vi "mecanum encoder read.vi"() -> ()   [LabVIEW 2014]
uses:
  global variables/devrefs.vi
panel:
  out "X Rate":dbl
  out "Y Rate":dbl
  in  "Reset Encoders":bool
  out "Y Distance":dbl
  out "X Distance":dbl
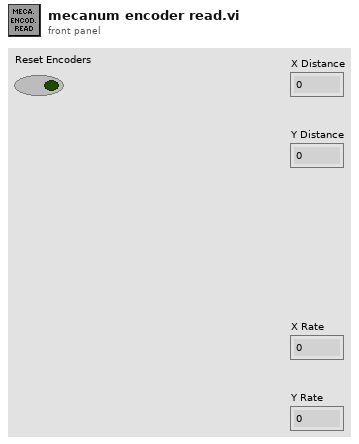
[diagram p1: front panel]
types:
  T1 = typedef "WPI_EncoderDevRef.ctl" = cluster{"DevStatus":errorcluster, "EncoderIndex":T2, "CounterIndex":T3, "DistancePerCount":dbl, "Decoding Type":T4}
  T2 = typedef "FPGA_EncoderIdx.ctl" = enum8{"Enc 0", "Enc 1", "Enc 2", "Enc 3", "Enc 4", "Enc 5", "Enc 6", "Enc 7", "Invalid"}
  T3 = typedef "FPGA_CounterCtrSystemIndex.ctl" = enum8{"Ctr 0", "Ctr 1", "Ctr 2", "Ctr 3", "Ctr 4", "Ctr 5", "Ctr 6", "Ctr 7", "Invalid"}
  T4 = typedef "WPI_EncoderType.ctl" = enum16{"1x", "2x", "4x"}
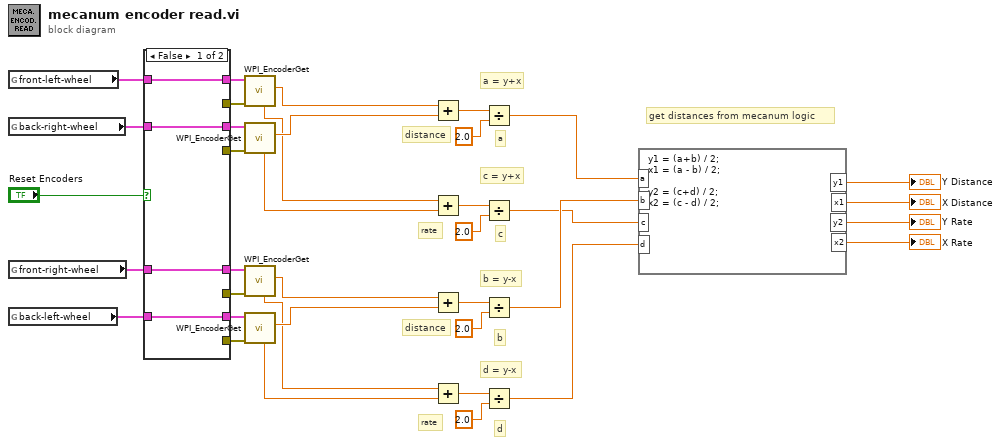
[diagram p0: block diagram]
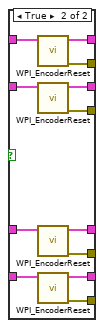
[diagram p2: hidden frame]
diagram:
  # "get distances from mecanum logic"
  # "distance"
  # "distance"
  # "rate"
  # "rate"
  # "c"
  # "c = y+x"
  # "d"
  # "d = y-x"
  # "b"
  # "a"
  # "b = y-x"
  # "a = y+x"
  n1 = global read "devrefs.vi" "front-left-wheel"() -> (w24:T1)
  n2 = global read "devrefs.vi" "back-right-wheel"() -> (w25:T1)
  n3 = global read "devrefs.vi" "front-right-wheel"() -> (w23:T1)
  n4 = global read "devrefs.vi" "back-left-wheel"() -> (w22:T1)
  n5 = case shown="False" "Reset Encoders" {
    tunnel: w25 -> [w40 w49]
    tunnel: w24 -> [w41 w52]
    tunnel: w23 -> [w39 w46]
    tunnel: w22 -> [w38 w43]
    tunnel: [w41 w53] -> w20
    tunnel: [w40 w50] -> w19
    tunnel: [w39 w47] -> w18
    tunnel: [w38 w44] -> w17
    tunnel: [_ w51] -> w16
    tunnel: [_ w48] -> w15
    tunnel: [_ w45] -> w14
    tunnel: [_ w42] -> w13
    frame False {
    }
    frame True {
      n6 = call <vilib>:"WPI_EncoderReset.vi"("EncoderDevRef"=w52) -> ("error out"=w51:errorcluster, "EncoderDevRef"=w53:T1)  [unwired: 9 in]
      n7 = call <vilib>:"WPI_EncoderReset.vi"("EncoderDevRef"=w49) -> ("error out"=w48:errorcluster, "EncoderDevRef"=w50:T1)  [unwired: 9 in]
      n8 = call <vilib>:"WPI_EncoderReset.vi"("EncoderDevRef"=w46) -> ("error out"=w45:errorcluster, "EncoderDevRef"=w47:T1)  [unwired: 9 in]
      n9 = call <vilib>:"WPI_EncoderReset.vi"("EncoderDevRef"=w43) -> ("error out"=w42:errorcluster, "EncoderDevRef"=w44:T1)  [unwired: 9 in]
    }
  }
  n10 = call <vilib>:"WPI_EncoderGet.vi"("error in (no error)"=w16, "EncoderDevRef"=w20) -> ("Distance"=w29:dbl, "Rate"=w6:dbl)  [unwired: 4 in, 4 out]
  n11 = call <vilib>:"WPI_EncoderGet.vi"("error in (no error)"=w15, "EncoderDevRef"=w19) -> ("Distance"=w28:dbl, "Rate"=w5:dbl)  [unwired: 4 in, 4 out]
  n12 = call <vilib>:"WPI_EncoderGet.vi"("error in (no error)"=w14, "EncoderDevRef"=w18) -> ("Distance"=w27:dbl, "Rate"=w10:dbl)  [unwired: 4 in, 4 out]
  n13 = call <vilib>:"WPI_EncoderGet.vi"("error in (no error)"=w13, "EncoderDevRef"=w17) -> ("Distance"=w26:dbl, "Rate"=w9:dbl)  [unwired: 4 in, 4 out]
  n14 = Add(x=w29, y=w28) -> (x+y=w37:dbl)
  n15 = Add(x=w6, y=w5) -> (x+y=w7:dbl)
  n16 = Add(x=w27, y=w26) -> (x+y=w34:dbl)
  n17 = Add(x=w10, y=w9) -> (x+y=w12:dbl)
  n18 = Divide(x=w37, y=2.0) -> (x/y=w33:dbl)
  n19 = Divide(x=w7, y=2.0) -> (x/y=w4:dbl)
  n20 = Divide(x=w34, y=2.0) -> (x/y=w32:dbl)
  n21 = Divide(x=w12, y=2.0) -> (x/y=w3:dbl)
  n22 = formula code="y1 = (a+b) / 2;\nx1 = (a - b) / 2;\n\ny2 = (c+d) / 2;\nx2 = (c - d) / 2;"("a"=w33, "b"=w32, "c"=w4, "d"=w3) -> ("y1"=→"Y Distance":dbl, "x1"=→"X Distance":dbl, "y2"=→"Y Rate":dbl, "x2"=→"X Rate":dbl)
